vi "_checkUnicode.vi"(8 "error in (no error)":errorcluster, 10 "String In":string, 11 "tJSONParser in":refnum<class "tJSONParser.lvclass">) -> (0 "error out":errorcluster, 3 "tJSONParser out":refnum<class "tJSONParser.lvclass">)   [LabVIEW 2013, in "JSON.lvlib" / "tJSONParser.lvclass"]
doc: "Validates that a unicode sequence does not contain any control codes."
uses:
  tJSONParser.lvclass
  _error.ctl
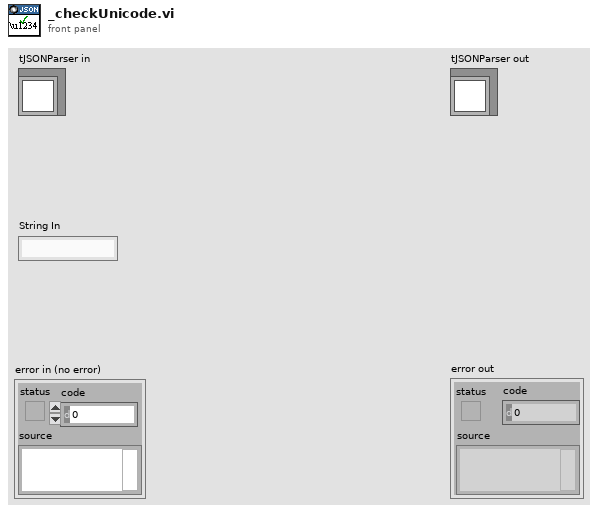
[diagram p1: front panel]
types:
  T1 = typedef "JSON.lvlib/tJSONParser.lvclass/_error.ctl" = enum16{"Missing Object Open", "Missing Pair Separator", "Missing Object End Or Separator", "Missing Pair String", "Unexpected Token", "Missing Array End Or Separator", "Invalid Escape Sequence", "Unexpected End Of File", "Invalid Unicode", "Unexpected End Of Line", "Invalid Numerical Constant"}
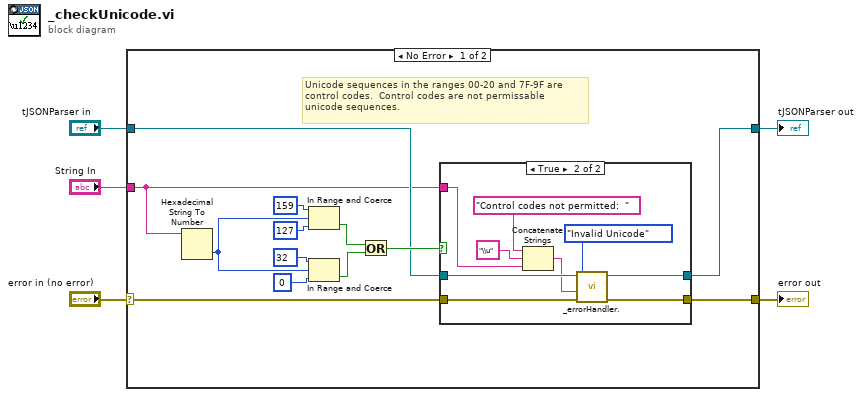
[diagram p0: block diagram]
diagram:
  n1 = case shown="No Error" "error in (no error)" {
    selector: "error in (no error)" -> [w10 w31]
    tunnel: [w11 w31] -> w4
    tunnel: [w7 w30] -> w2
    tunnel: "tJSONParser in" -> [w8 w30]
    tunnel: "String In" -> [w6 _]
    frame No Error {
      # "Unicode sequences in the ranges 00-20 and 7F-9F are \ncontrol codes.  Control codes are not permissable \nunicode sequences."
      n2 = Hexadecimal String To Number(string=w6) -> (number=w14:u32)  [unwired: 2 in, 1 out]
      n3 = In Range and Coerce(upper limit=u32 159, x=w14, lower limit=u32 127 ("upper limit")) -> (In Range?=w13:bool)  [unwired: 1 out]
      n4 = In Range and Coerce(upper limit=u32 32, x=w14, lower limit=u32 0 ("upper limit")) -> (In Range?=w12:bool)  [unwired: 1 out]
      n5 = Or(x=w13, y=w12) -> (x .or. y?=w9:bool)
      n6 = case shown="True" w9 {
        tunnel: [w19 w27] -> w11
        tunnel: w10 -> [w19 w28]
        tunnel: w8 -> [w20 w26]
        tunnel: [w20 w25] -> w7
        tunnel: w6 -> [_ w22]
        frame False {
        }
        frame True {
          n7 = Concatenate Strings("Control codes not permitted:  " ("string"), "\\u" ("string"), w22) -> (w24:string)
          n8 = call "_errorHandler..vi"("error in (no error)"=w28, "Additional Text"=w24, "Error Type"=_error."Invalid Unicode", "JSON Parser In"=w26) -> ("error out"=w27:errorcluster, "JSON Parser Out"=w25:refnum<class "tJSONParser.lvclass">)  [unwired: 6 in]
        }
      }
    }
    frame Error {
    }
  }
  "error out" <- w4
  "tJSONParser out" <- w2
